vi "EVENT.vi"(4 "用户参数":T1, 5 "事件数据":cluster{"uiMsg":refnum<k7>, "cancel":bool}, 6 "控件引用":refnum<k7>, 7 "事件通用数据":cluster{"事件源":i32, "事件类型":u32, "时间标识":u32}) -> (1 "事件数据输出":cluster{"cancel":bool})   [LabVIEW 2013]
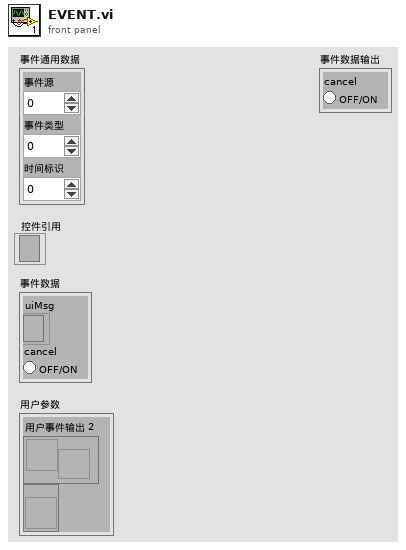
[diagram p1: front panel]
types:
  T1 = cluster{"用户事件输出 2":refnum<user-event>, refnum<vi>}
  T2 = cluster{"Event":i32, "ActiveXData":variant, "NumericData":dbl}
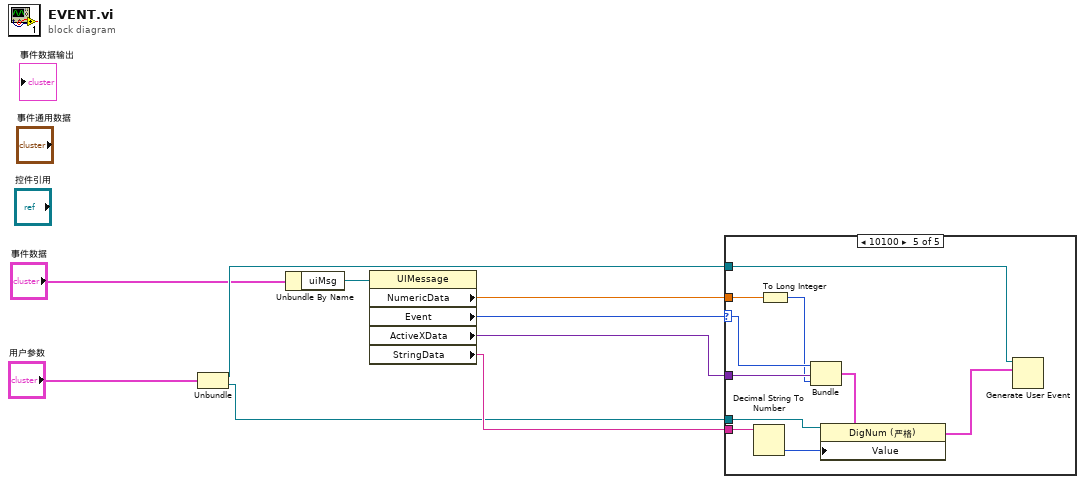
[diagram p0: block diagram]
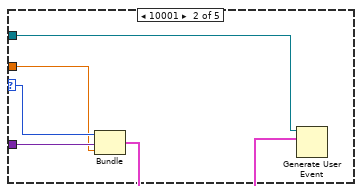
[diagram p3: hidden frame]
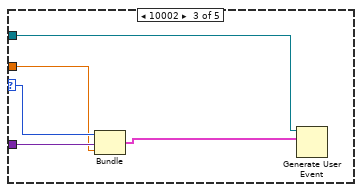
[diagram p4: hidden frame]
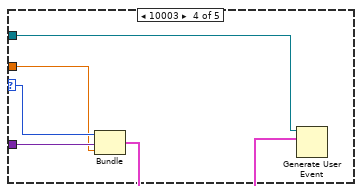
[diagram p5: hidden frame]
diagram:
  n1 = Unbundle("用户参数") -> ("用户事件输出 2"=w5:refnum<user-event>, w1:refnum<vi>)
  n2 = Unbundle By Name("事件数据") -> ("uiMsg"=w9:refnum<k7>)
  n3 = property class="UIMessage"(reference=w9) -> ("NumericData"=w3:dbl, "Event"=w8:i32, "ActiveXData"=w7:variant, "StringData"=w2:string)  [unwired: 1 in, 2 out]
  n4 = case shown="10100" w8 {
    selector: w8 -> [_ w14 w19 w24 w33]
    tunnel: w7 -> [_ w11 w18 w23 w32]
    tunnel: w5 -> [_ w12 w16 w21 w30]
    tunnel: w3 -> [_ w10 w15 w20 w29]
    tunnel: w2 -> [_ _ _ _ w26]
    tunnel: w1 -> [_ _ _ _ w25]
    frame 0, Default {
    }
    frame 10001 {
      n5 = Bundle("Event"=w14, "ActiveXData"=w11, "NumericData"=w10) -> (w13:T2)  [unwired: 1 in]
      n6 = Generate User Event(user event=w12, event data cluster=w13) -> ()  [unwired: 2 in, 2 out]
    }
    frame 10002 {
      n7 = Bundle("Event"=w19, "ActiveXData"=w18, "NumericData"=w15) -> (w17:T2)  [unwired: 1 in]
      n8 = Generate User Event(user event=w16, event data cluster=w17) -> ()  [unwired: 2 in, 2 out]
    }
    frame 10003 {
      n9 = Bundle("Event"=w24, "ActiveXData"=w23, "NumericData"=w20) -> (w22:T2)  [unwired: 1 in]
      n10 = Generate User Event(user event=w21, event data cluster=w22) -> ()  [unwired: 2 in, 2 out]
    }
    frame 10100 {
      n11 = Decimal String To Number(string=w26) -> (number=w27:i32)  [unwired: 2 in, 1 out]
      n12 = To Long Integer(number=w29) -> (32bit integer=w28:i32)
      n13 = Bundle("Event"=w33, "ActiveXData"=w32, w28) -> (w31:cluster{"Event":i32, "ActiveXData":variant, i32})  [unwired: 1 in]
      n14 = property class="DigNum (严格)"(reference=w25, "Value"=w27) -> ()  [unwired: 1 in, 2 out]
      n15 = Generate User Event(user event=w30, event data cluster=w31) -> ()  [unwired: 2 in, 2 out]
    }
  }
